vi "configREF_f.vi"(7 "address":string, 8 "error in (no error)":errorcluster, 9 "new f (Hz)":dbl, 10 "lockin Channel":T1=1 min=1 max=16, 11 "Channels: Lockin":T2={"REF f (Hz)"=[13.0], "REF phi (°)"=[0.0]} {"REF phi (°)" format="%#_3g"}) -> (0 "error out":errorcluster, 3 "Channels: Lockin":T2={"REF f (Hz)"=[13.0], "REF phi (°)"=[0.0]} {"REF phi (°)" format="%#_3g"})   [LabVIEW 2016]
doc: "API to configure a REF frequency.\n\nSpecify which channel you want to change and the value you want to set.\n\nIf address=\"\", this API reads from localhost\nIf address is remote lockin, you need to add this computer to allowed whitelist on the lockin computer you are trying to access."
uses:
  Typedefs/REF-cluster.ctl
  Typedefs/REF_f-array.ctl
  Typedefs/REF_phi-array.ctl
  Typedefs/REF_Channel-Numeric.ctl
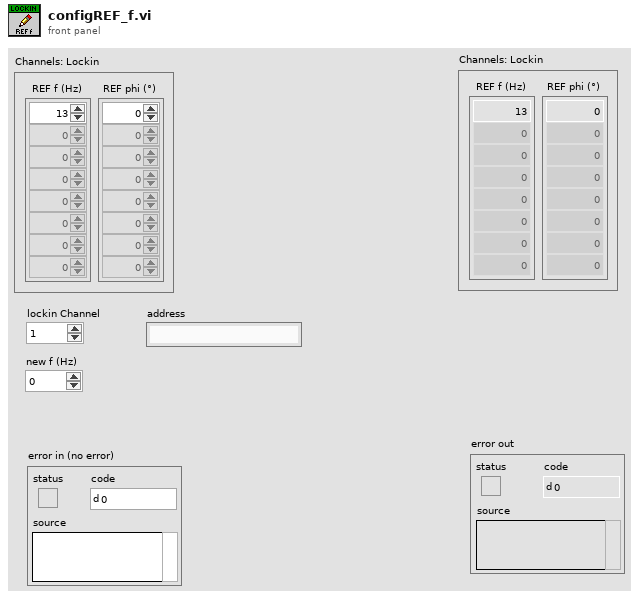
[diagram p1: front panel]
types:
  T1 = typedef "REF_Channel-Numeric.ctl" = i32
  T2 = typedef "REF-cluster.ctl" = cluster{"REF f (Hz)":T3, "REF phi (°)":T4}
  T3 = typedef "REF_f-array.ctl" = dbl[]
  T4 = typedef "REF_phi-array.ctl" = dbl[]
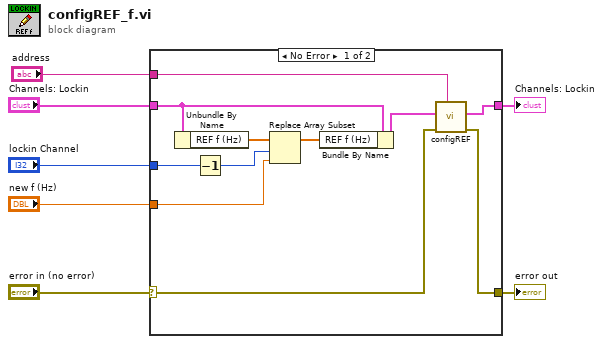
[diagram p0: block diagram]
diagram:
  n1 = case shown="No Error" "error in (no error)" {
    selector: "error in (no error)" -> [w13 w20]
    tunnel: "Channels: Lockin" -> [w16 w19]
    tunnel: [w8 w19] -> w6
    tunnel: "lockin Channel" -> [w15 _]
    tunnel: "new f (Hz)" -> [w14 _]
    tunnel: [w12 w20] -> w2
    tunnel: "address" -> [w11 _]
    frame No Error {
      n2 = Unbundle By Name(w16) -> ("REF f (Hz)"=w17:T3)
      n3 = Decrement(x=w15) -> (x-1=w10:T1)
      n4 = Replace Array Subset(array=w17, new element=w14, index=w10) -> (w18:T3)
      n5 = Bundle By Name(cluster=w16, "REF f (Hz)"=w18) -> (w9:T2)
      n6 = call "configREF.vi"("address"=w11, "error in (no error)"=w13, "Channels: Lockin in"=w9) -> ("error out"=w12:errorcluster, "Channels: Lockin out"=w8:T2)  [unwired: 7 in]
    }
    frame Error {
    }
  }
  "Channels: Lockin" <- w6
  "error out" <- w2
